vi "游戏是否胜利.vi"(1 "地图":i32[][](array[numeric])) -> (0 "胜利":bool)   [LabVIEW 2017]
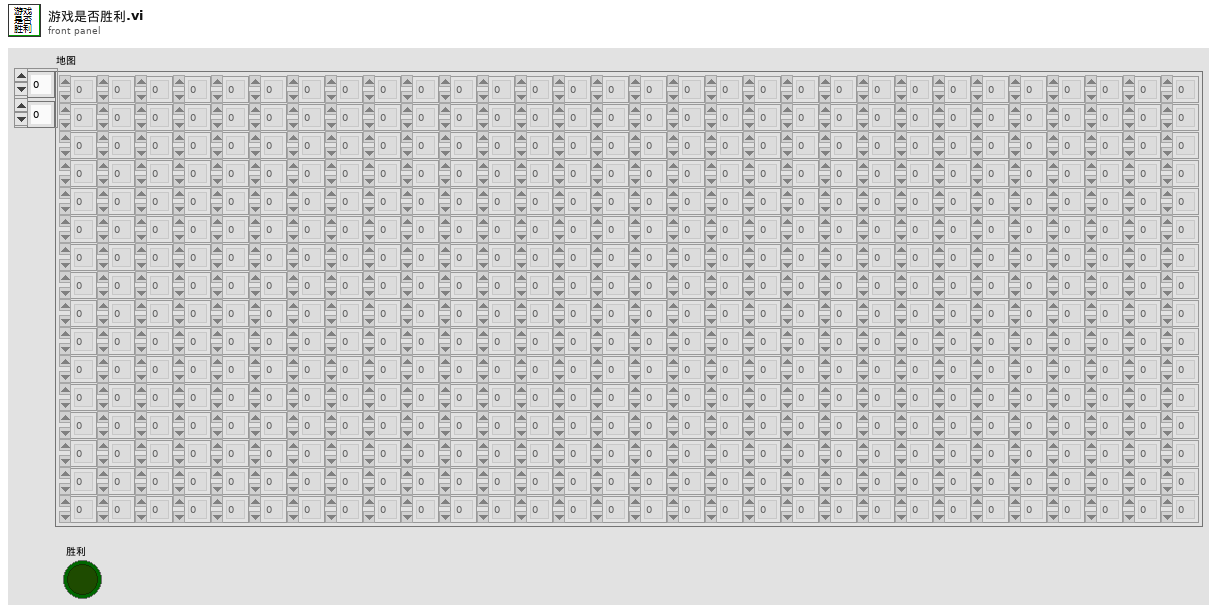
[diagram p1: front panel]
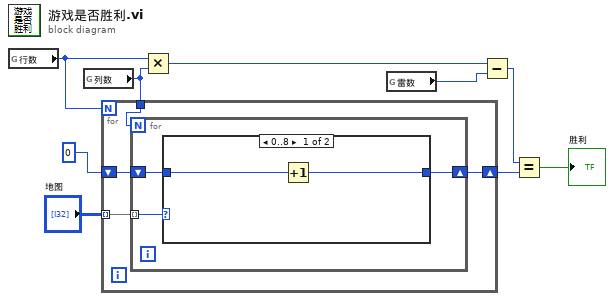
[diagram p0: block diagram]
diagram:
  n1 = global read "全局变量.vi" "行数"() -> (w1:i32)
  n2 = global read "全局变量.vi" "列数"() -> (w2:i32)
  n3 = for {
    N: w1 -> [_]
    tunnel: "地图" -> [w13] mode=indexing
    shift-right: [w11] -> w6
    shift-left: 0 -> [w12]
    tunnel: w2 -> [w10]
    n4 = for {
      N: w10 -> [_]
      tunnel: w13 -> [w16] mode=indexing
      shift-right: [w14] -> w11
      shift-left: w12 -> [w15]
      n5 = case shown="0..8" w16 {
        tunnel: w15 -> [w18 w19]
        tunnel: [w17 w19] -> w14
        frame 0..8 {
          n6 = Increment(x=w18) -> (x+1=w17:i32)
        }
        frame 9..16, Default {
        }
      }
    }
  }
  n7 = Multiply(x=w1, y=w2) -> (x*y=w5:i32)
  n8 = global read "全局变量.vi" "雷数"() -> (w4:i32)
  n9 = Subtract(x=w5, y=w4) -> (x-y=w3:i32)
  n10 = Equal?(x=w3, y=w6) -> (x = y?=→"胜利":bool)
